vi "Update Frame Array.vi"(6 "Field Size":refnum<class "Field.lvclass">, 7 "Balls":refnum<class "Ball.lvclass">[](array[class]), 8 "max ball vel":dbl, 9 "Fps":dbl=40.0, 10 "Detection Frame in":refnum<class "Camera.lvclass">[](array[class]), 11 "Array Detection Frame in":refnum<class "Camera.lvclass">[](array[class])) -> (2 "sum":i32, 3 "Detection Frame out":refnum<class "Camera.lvclass">[](array[class]))   [LabVIEW 2018]
uses:
  Controls/SSL Detection Frame.ctl
  Controls/SSL Detection Robot.ctl
  <vilib>/Analysis/Matrix/Datatypes/RealMatrix.ctl
  Controls/SSL Detection Ball.ctl
  Camera_class/Camera.lvclass
  Field_class/Field.lvclass
  Ball_class/Ball.lvclass
  <vilib>/Analysis/Matrix/NI_Matrix.lvlib
panel:
  out "Array":T1[](array[typedef]) {"robots_blue"."height" format="%+4.3f"; "robots_blue"."pixel_y" format="%+4.3f"; "robots_blue"."pixel_x" format="%+4.3f"; "robots_blue"."orientation" format="%+4.3f"; "robots_blue"."y" format="%+4.3f"; "robots_blue"."confidence" format="%4.3f"; "robots_blue"."x" format="%+4.3f"; "robots_yellow"."height" format="%+4.3f"; "robots_yellow"."pixel_y" format="%+4.3f"; "robots_yellow"."pixel_x" format="%+4.3f"; "robots_yellow"."orientation" format="%+4.3f"; "robots_yellow"."y" format="%+4.3f"; "robots_yellow"."confidence" format="%4.3f"; "robots_yellow"."x" format="%+4.3f"}
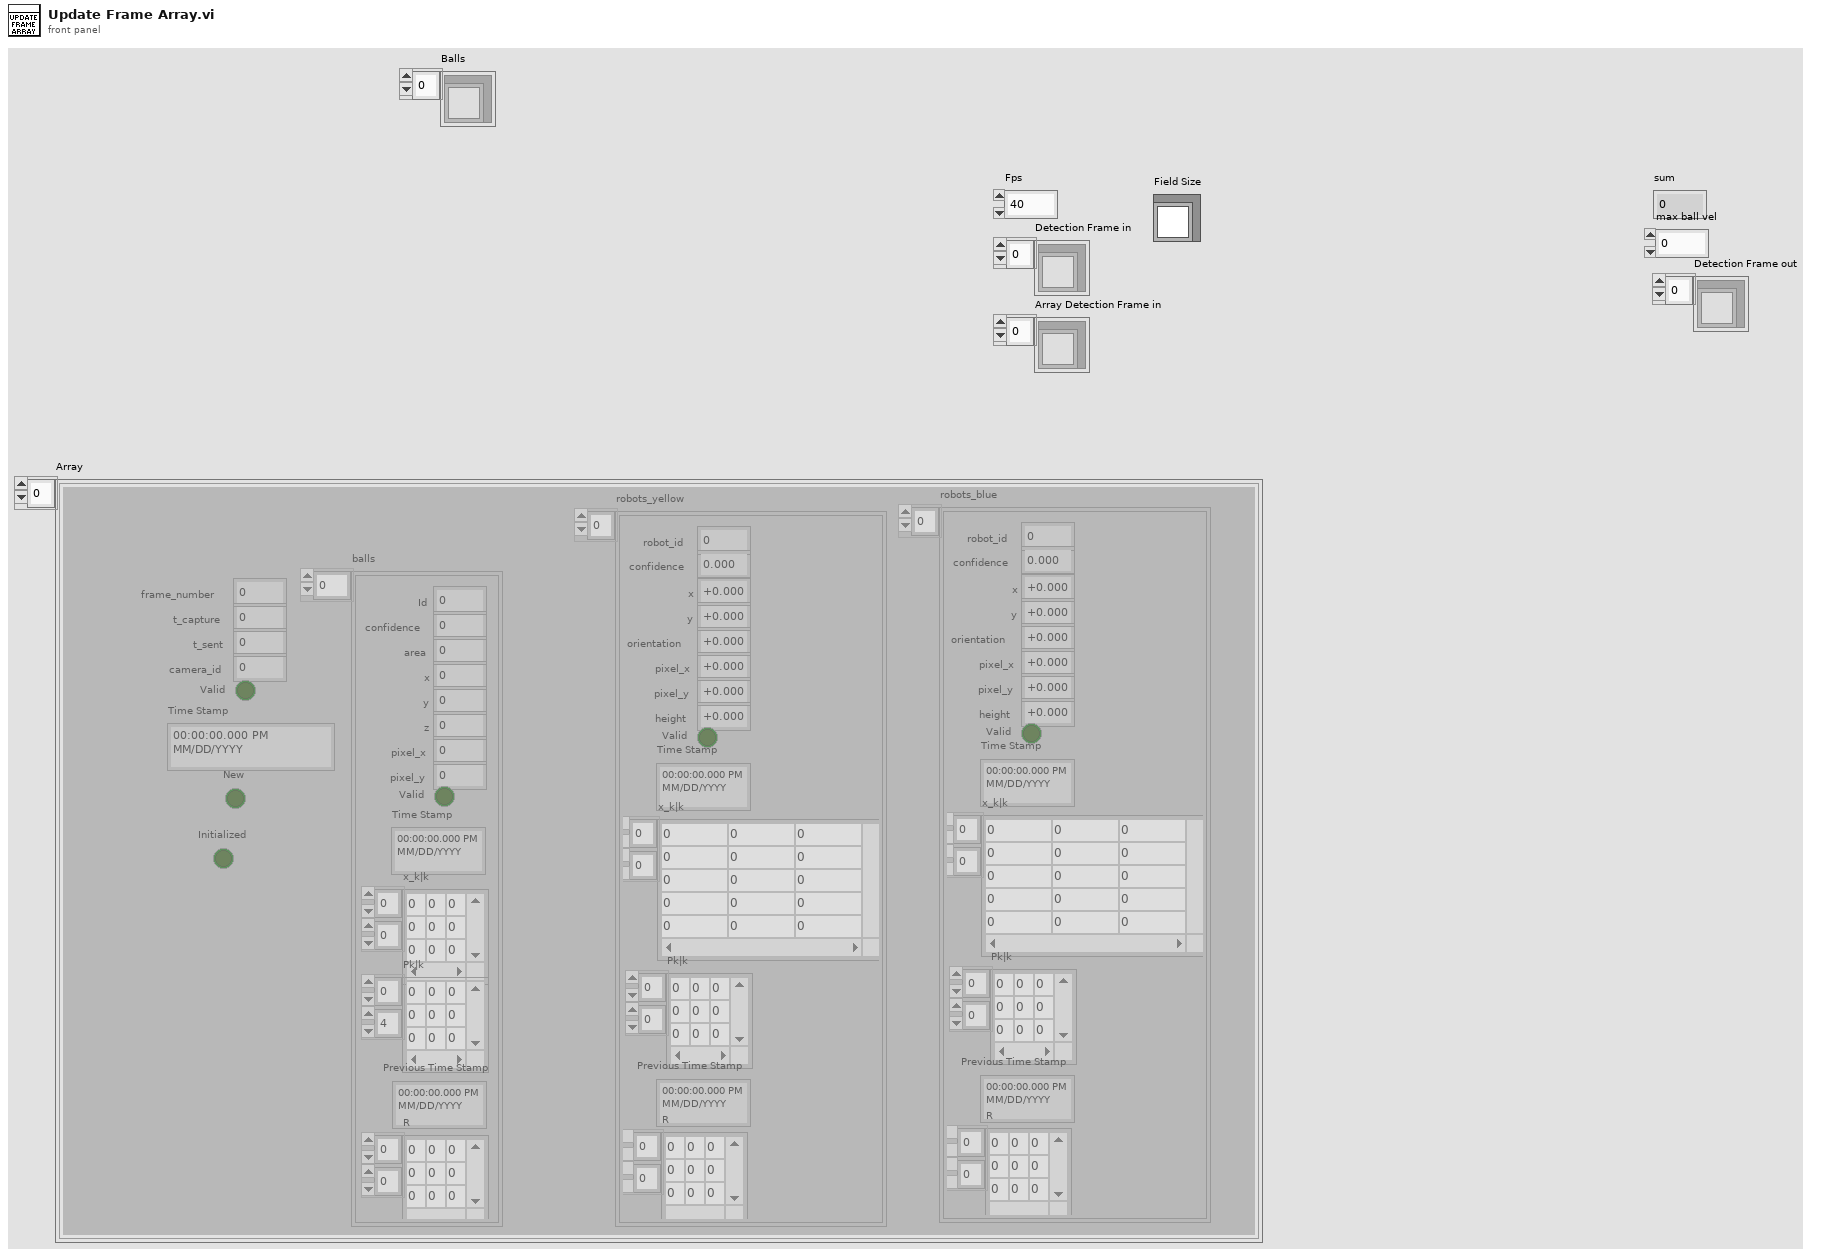
[diagram p1: front panel]
types:
  T1 = typedef "SSL Detection Frame.ctl" = cluster{"frame_number":u32, "t_capture":dbl, "t_sent":dbl, "camera_id":u32, "robots_yellow":T2[], "robots_blue":T2[], "balls":T4[], "Valid":bool, "Time Stamp":timestamp, "New":bool, "Initialized":bool}
  T2 = typedef "SSL Detection Robot.ctl" = cluster{"x":sgl, "robot_id":u32, "confidence":sgl, "y":sgl, "orientation":sgl, "pixel_x":sgl, "pixel_y":sgl, "height":sgl, "Valid":bool, "Time Stamp":timestamp, "x_k|k":T3, "Pk|k":T3, "Previous Time Stamp":timestamp, "R":T3}
  T3 = typedef "NI_Matrix.lvlib/RealMatrix.ctl" = dbl[][]
  T4 = typedef "SSL Detection Ball.ctl" = cluster{"x":sgl, "area":u32, "confidence":sgl, "y":sgl, "z":sgl, "pixel_x":sgl, "pixel_y":sgl, "Valid":bool, "Time Stamp":timestamp, "x_k|k":T3, "Pk|k":T3, "Id":u32, "Previous Time Stamp":timestamp, "R":T3}
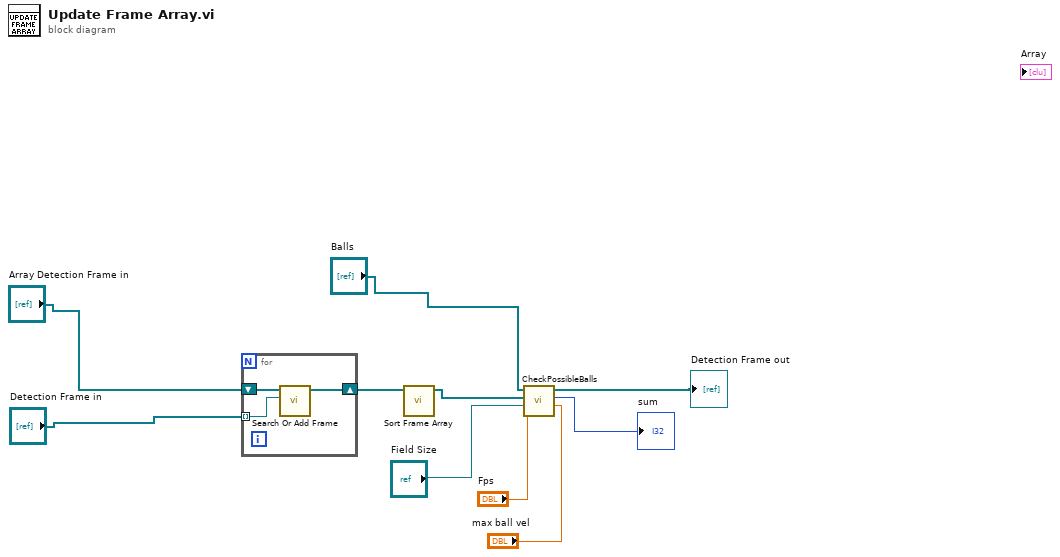
[diagram p0: block diagram]
diagram:
  n1 = for {
    tunnel: "Detection Frame in" -> [w12] mode=indexing
    shift-right: [w13] -> w10
    shift-left: "Array Detection Frame in" -> [w11]
    n2 = call "Search Or Add Frame.vi"("Detection Frame in 3"=w12, "Detection Frame in 4"=w11) -> ("Detection Frame in 5"=w13:refnum<class "Camera.lvclass">[])  [unwired: 9 in]
  }
  n3 = call "Sort Frame Array.vi"("Detection Frame In in"=w10) -> ("Array"=w6:refnum<class "Camera.lvclass">[])  [unwired: 10 in]
  n4 = call "CheckPossibleBalls.vi"("max ball vel"="max ball vel", "Fps"="Fps", "Field Size"="Field Size", "Array of cameras"=w6, "last ball choosed by mediacameras"="Balls") -> ("sum"=→"sum":i32, "Detection Frame In out"=→"Detection Frame out":refnum<class "Camera.lvclass">[])  [unwired: 5 in]
